vi "Write currentTimeToObservable_min.vi"(8 "error in (no error)":errorcluster, 10 "currentTimeToObservable_min":dbl[unit], 11 "Limits in":refnum<class "Limits.lvclass">) -> (0 "error out":errorcluster, 3 "Limits out":refnum<class "Limits.lvclass">)   [LabVIEW 2014, in "TCSDataDefinitions.lvlib" / "TCSPublicStatus.lvlib" / "Limits.lvlib" / "Limits.lvclass"]
uses:
  Limits.lvclass
  Limits.lvclass/Limits.ctl
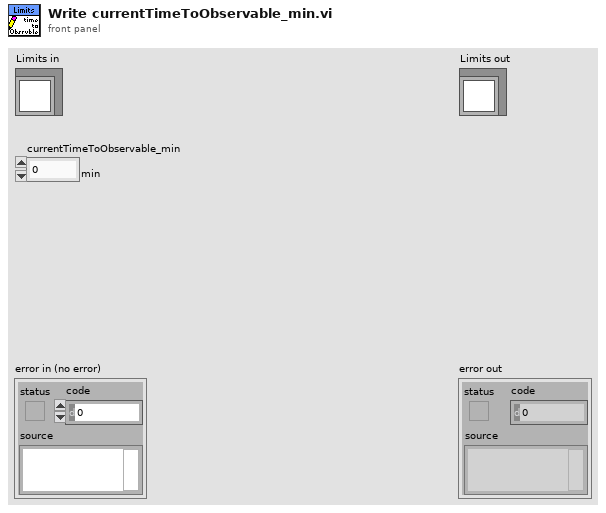
[diagram p1: front panel]
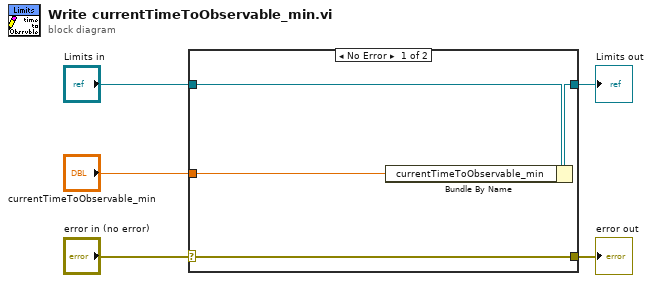
[diagram p0: block diagram]
diagram:
  n1 = case shown="No Error" "error in (no error)" {
    selector: "error in (no error)" -> [w9 w10]
    tunnel: [w9 w10] -> w4
    tunnel: [w7 w11] -> w2
    tunnel: "Limits in" -> [w8 w11]
    tunnel: "currentTimeToObservable_min" -> [w6 _]
    frame No Error {
      n2 = Bundle By Name(cluster=w8, "currentTimeToObservable_min"=w6) -> (w7:refnum<class "Limits.lvclass">)
    }
    frame Error {
    }
  }
  "error out" <- w4
  "Limits out" <- w2
